vi "Set Ext Clock.vi"(7 "Requested state of Ext clock":bool, 11 "machine":T1 {"TimeStamp" format="%.2f"}) -> (0 "error out":errorcluster, 3 "Reply data":string)   [LabVIEW 2020]
uses:
  DataSocketCluster external.ctl
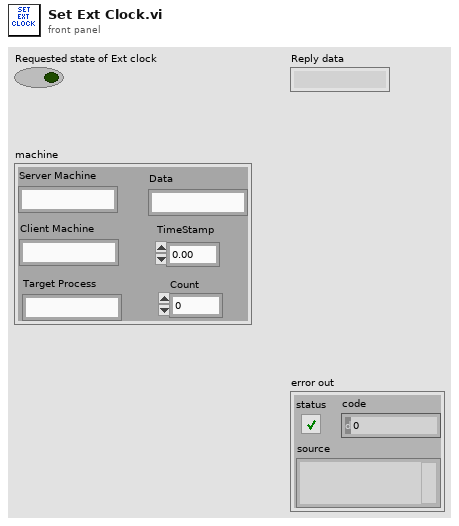
[diagram p1: front panel]
types:
  T1 = typedef "DataSocketCluster external.ctl" = cluster{"Server Machine":string, "Client Machine":string, "Data":string, "TimeStamp":dbl, "Count":i32, "Target Process":string}
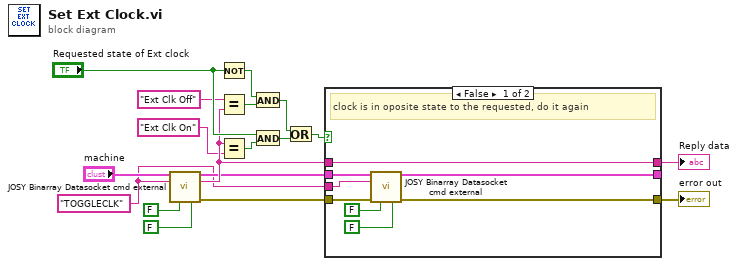
[diagram p0: block diagram]
diagram:
  w1 = "TOGGLECLK" ("Command")
  n1 = call "JOSY Binarray Datasocket cmd external.vi"("DataSocketCluster In"="machine", "Command"=w1, "Command has variable"=FALSE, "String"=FALSE) -> ("DataSocketCluster Out"=w8:T1, "Reply data"=w13:string, "error out"=w17:errorcluster)  [unwired: 8 in, 1 out]
  n2 = Not(x="Requested state of Ext clock") -> (.not. x?=w14:bool)
  n3 = Equal?(x="Ext Clk Off" ("Reply data"), y=w13) -> (x = y?=w10:bool)
  n4 = Equal?(x=w13, y="Ext Clk On" ("Reply data")) -> (x = y?=w6:bool)
  n5 = And(x=w14, y=w10) -> (x .and. y?=w11:bool)
  n6 = And(x="Requested state of Ext clock", y=w6) -> (x .and. y?=w9:bool)
  n7 = Or(x=w11, y=w9) -> (x .or. y?=w16:bool)
  n8 = case shown="False" w16 {
    tunnel: [w20 w29] -> w7
    tunnel: w13 -> [w20 w29]
    tunnel: w8 -> [w24 w28]
    tunnel: [w23 w28] -> _
    tunnel: w17 -> [w22 w27]
    tunnel: [w21 w27] -> w18
    tunnel: w1 -> [w19 _]
    frame False {
      # "clock is in oposite state to the requested, do it again"
      n9 = call "JOSY Binarray Datasocket cmd external.vi"("DataSocketCluster In"=w24, "Command"=w19, "error in (no error)"=w22, "Command has variable"=FALSE, "String"=FALSE) -> ("DataSocketCluster Out"=w23:T1, "error out"=w21:errorcluster)  [unwired: 7 in, 2 out]
    }
    frame True {
      # "clock is as user wanted, nothing to do"
    }
  }
  "error out" <- w18
  "Reply data" <- w7
